vi "电源管理UI.vi"() -> ()   [LabVIEW 2016, in "PLC.lvlib"]
uses:
  PLC.lvlib
  <vilib>/Utility/miscctls.llb/LVPointTypeDef.ctl
  <vilib>/ptbypt/NI_PtbyPt.lvlib
panel:
  in  "电源控制":T1
  in  "副屏看门狗启用":u16(ring) caption="副屏看门狗启用：" items=["关闭", "打开"]
  in  "副屏看门狗设置":u16 caption="副屏看门狗设置："
  out "副屏看门狗计时":u16 caption="副屏看门狗计时："
  in  "主屏看门狗启用":u16(ring) caption="主屏看门狗启用：" items=["关闭", "打开"]
  in  "主屏看门狗设置":u16 caption="主屏看门狗设置："
  out "主屏看门狗计时":u16 caption="主屏看门狗计时："
  out "漏电报警累加值":u16 caption="漏电报警累加值："
  out "外部电源状态":u16(ring) caption="外部电源状态：" items=["正常", "异常"]
  out "当前报警状态":u16(ring) caption="当前报警状态：" items=["无报警"=0, "过压报警"=1, "欠压报警"=2, "过流报警"=4, "漏电报警"=8]
  out "通讯状态":u16(ring) caption="通讯状态：" items=["正常", "异常"]
  out "内部电源状态":u16(ring) caption="内部电源状态：" items=["异常", "正常"]
  out "过流报警累加值":u16 caption="过流报警累加值："
  out "欠压报警累加值":u16 caption="欠压报警累加值："
  out "过压报警累加值":u16 caption="过压报警累加值："
  out "当前漏电电流":dbl caption="当前漏电电流："
  out "当前电流":dbl caption="当前电流："
  out "当前电压":u16 caption="当前电压："
  # "s"
  # "s"
  # "s"
  # "s"
  # "mA"
  # "A"
  # "V"
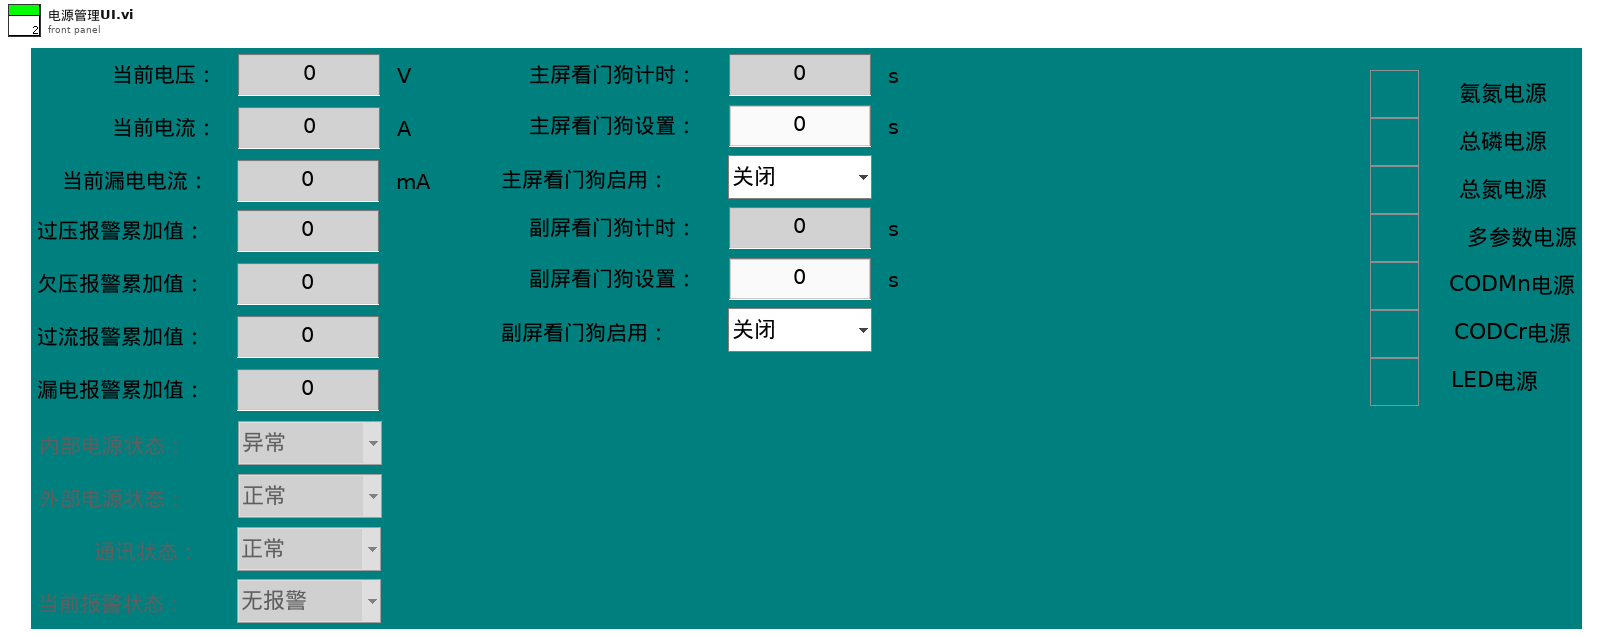
[diagram p1: front panel]
types:
  T1 = cluster{"氨氮电源":bool, "总磷电源":bool, "总氮电源":bool, "多参数电源":bool, "CODMn电源":bool, "CODCr电源":bool, "LED电源":bool}
  T2 = typedef "LVPointTypeDef.ctl" = cluster{"Horizontal":i16, "Vertical":i16}
  T3 = cluster{"R0":i16, "R1":i16, "R2":i16, "R3":i16, "R4":i16, "R5":i16, "R6":i16, "R7":i16, "R8":i16, "R9":i16, "R10":i16, "R11":i16, "R12":i16, "R13":i16, "R14":i16, "R15":i16, "R16":i16, "R17":i16, "R18":i16, "R19":i16, "R20":i16, "R21":i16, "R22":i16, "R23":i16, "R24":i16, "R25":i16, "R26":i16, "R27":i16, "R28":i16, "R29":i16, "R30":i16, "R31":i16, "R32":i16, "R33":i16, "R34":i16, "R35":i16, "R36":i16, "R37":i16, "R38":i16, "R39":i16}
  T4 = cluster{"R100":i16, "R101":i16, "R102":i16, "R103":i16, "R104":i16, "R105":i16, "R106":i16, "R107":i16, "R108":i16, "R109":i16, "R110":i16, "R111":i16, "R112":i16, "R113":i16, "R114":i16, "R115":i16, "R116":i16, "R117":i16, "R118":i16, "R119":i16, "R120":i16}
  T5 = cluster{"命令":string, "数据":cluster{"starting address":u16, "holding register values":u16[]}}
  T6 = cluster{"命令":string, "数据":cluster{"starting address":u16, "holding register value":u16}}
  T7 = cluster{"时间标识":timestamp, "设备":string, "日志信息":string}
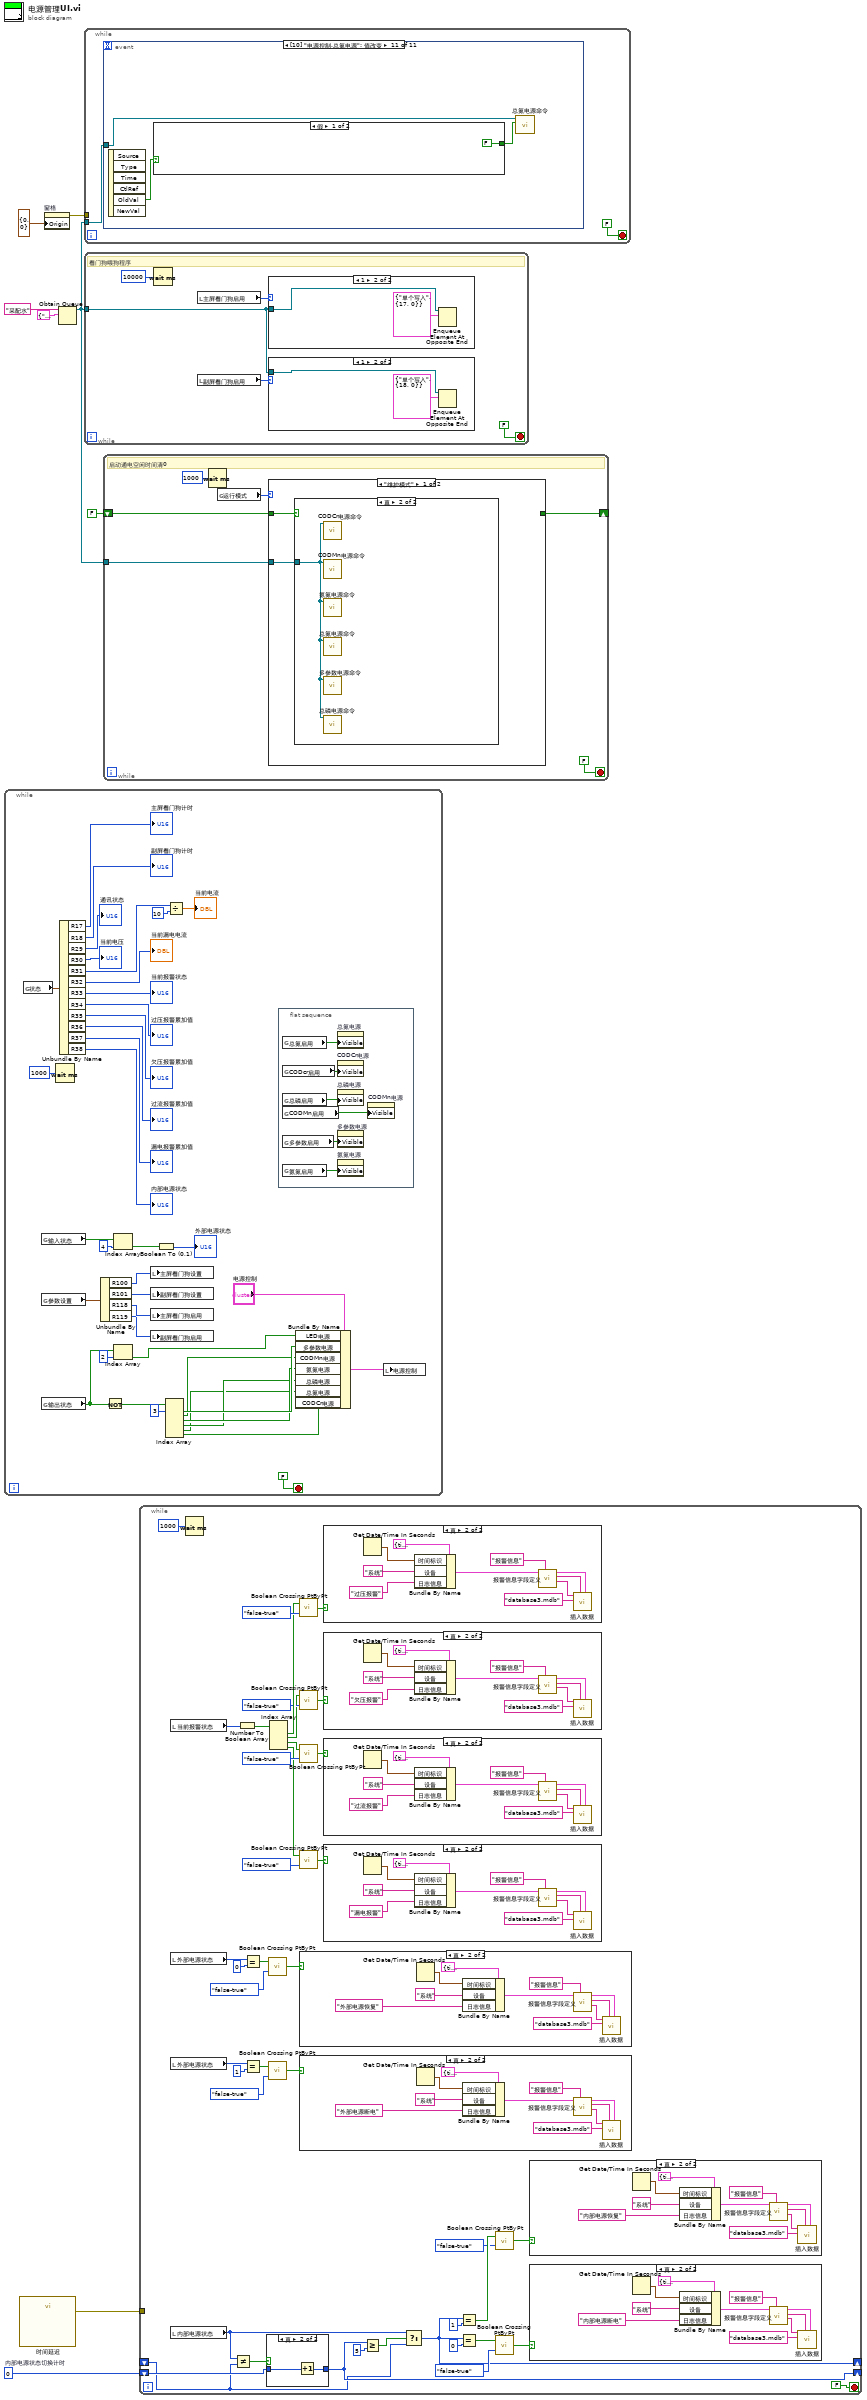
[diagram p0: block diagram]
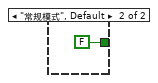
[diagram p14: hidden frame]
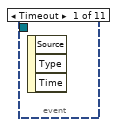
[diagram p15: hidden frame]
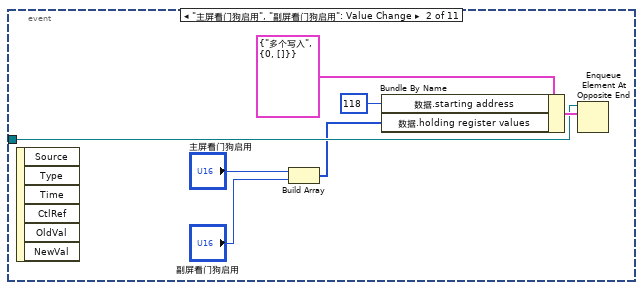
[diagram p16: hidden frame]
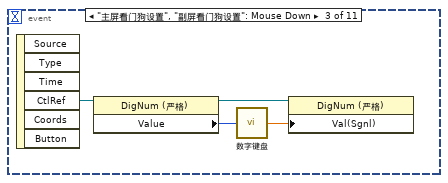
[diagram p17: hidden frame]
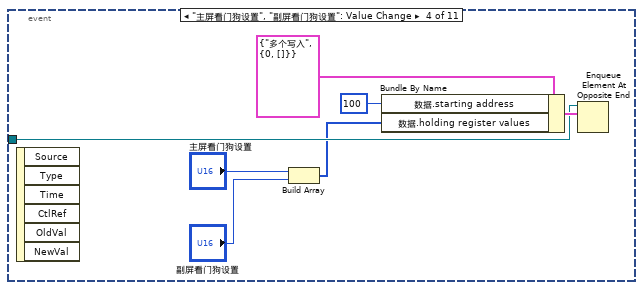
[diagram p18: hidden frame]
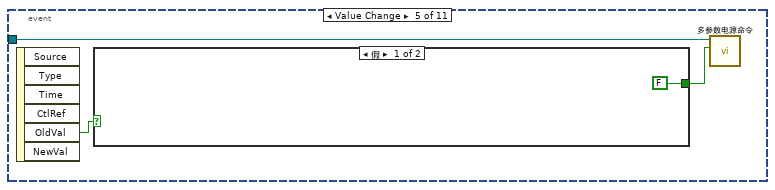
[diagram p19: hidden frame]
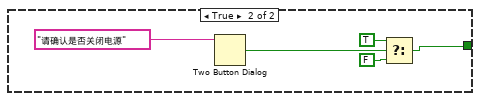
[diagram p20: hidden frame]
diagram:
  w1 = u16 0  # 内部电源状态切换计时
  n1 = while {
    stop <- FALSE stop-if-true
    n2 = global read "采配水全局变量.vi" "状态"() -> (w44:T3)
    n3 = global read "采配水全局变量.vi" "输入状态"() -> (w31:bool[])
    n4 = global read "采配水全局变量.vi" "参数设置"() -> (w25:T4)
    n5 = global read "采配水全局变量.vi" "输出状态"() -> (w19:bool[])
    n6 = Wait (ms)(milliseconds to wait=u32 1000 ("等待时间（毫秒）")) -> ()  [unwired: 1 out]
    n7 = Unbundle By Name(w44) -> ("R17"=→"主屏看门狗计时":i16, "R18"=→"副屏看门狗计时":i16, "R29"=→"通讯状态":i16, "R30"=→"当前电压":i16, "R31"=w41:i16, "R32"=→"当前漏电电流":i16, "R33"=→"当前报警状态":i16, "R34"=→"过压报警累加值":i16, "R35"=→"欠压报警累加值":i16, "R36"=→"过流报警累加值":i16, "R37"=→"漏电报警累加值":i16, "R38"=→"内部电源状态":i16)
    n8 = Unbundle By Name(w25) -> ("R100"=w24:i16, "R101"=w23:i16, "R118"=w22:i16, "R119"=w21:i16)
    n9 = Not(x=w19) -> (.not. x?=w45:bool[])
    n10 = Index Array(array=w31, index=4 ("索引")) -> (element=w29:bool)
    n11 = Index Array(array=w19, index=2 ("索引")) -> (element=w16:bool)
    n12 = local write "主屏看门狗设置"(w24) -> ()
    n13 = local write "副屏看门狗设置"(w23) -> ()
    n14 = local write "主屏看门狗启用"(w22) -> ()
    n15 = local write "副屏看门狗启用"(w21) -> ()
    n16 = Boolean To (0,1)(Boolean=w29) -> (0, 1=→"外部电源状态":i16)
    n17 = Index Array(array=w45, index #1=3 ("索引")) -> (element #1=w15:bool, element #2=w14:bool, element #3=w13:bool, element #4=w12:bool, element #5=w11:bool, element #6=w10:bool)  [unwired: 5 in]
    n18 = Divide(x=w41, y=i16 10) -> (x/y=→"当前电流":dbl)
    n19 = flat-sequence {
      frame #0 {
        n20 = global read "系统设置全局变量.vi" "总氮启用"() -> (w52:bool)
        n21 = global read "系统设置全局变量.vi" "CODcr启用"() -> (w49:bool)
        n22 = global read "系统设置全局变量.vi" "总磷启用"() -> (w48:bool)
        n23 = global read "系统设置全局变量.vi" "CODMn启用"() -> (w51:bool)
        n24 = global read "系统设置全局变量.vi" "多参数启用"() -> (w50:bool)
        n25 = global read "系统设置全局变量.vi" "氨氮启用"() -> (w53:bool)
        n26 = property on="总氮电源" class="Bool (严格)"("Visible"=w52) -> ()  [unwired: 2 in, 2 out]
        n27 = property on="CODCr电源" class="Bool (严格)"("Visible"=w49) -> ()  [unwired: 2 in, 2 out]
        n28 = property on="总磷电源" class="Bool (严格)"("Visible"=w48) -> ()  [unwired: 2 in, 2 out]
        n29 = property on="多参数电源" class="Bool (严格)"("Visible"=w50) -> ()  [unwired: 2 in, 2 out]
        n30 = property on="氨氮电源" class="Bool (严格)"("Visible"=w53) -> ()  [unwired: 2 in, 2 out]
        n31 = property on="CODMn电源" class="Bool (严格)"("Visible"=w51) -> ()  [unwired: 2 in, 2 out]
      }
    }
    n32 = Bundle By Name(cluster="电源控制", "LED电源"=w16, "多参数电源"=w15, "CODMn电源"=w14, "氨氮电源"=w13, "总磷电源"=w12, "总氮电源"=w11, "CODCr电源"=w10) -> (w9:T1)
    n33 = local write "电源控制"(w9) -> ()
  }
  n34 = call "时间延迟"() -> ("error out"=w3:errorcluster)  [unwired: 11 in]
  n35 = property on="窗格" class="Pane"("Origin"=T2 {"Horizontal"=0, "Vertical"=0} ("原点")) -> (error out=w5:errorcluster)  [unwired: 2 in, 1 out]
  n36 = Obtain Queue(name (unnamed)="采配水" ("名称（未命名）"), element data type=cluster{"命令":string, "数据":variant} {"命令"="", "数据"=variant}) -> (queue out=w2:refnum<queue>)  [unwired: 3 in, 2 out]
  n37 = while {
    tunnel: w2 -> [w54]
    tunnel: w5 -> [_]
    stop <- FALSE stop-if-true
    n38 = event shown="[10] \"电源控制.总氮电源\": 值改变" {
      selector: _ -> [_ _ _ _ _ _ _ _ _ _ _]
      dyn-events: _ -> [_ _ _ _ _ _ _ _ _ _ _]
      timeout: _ -> [_ _ _ _ _ _ _ _ _ _ _]
      tunnel: w54 -> [_ w59 _ w70 w76 w84 w94 w103 w112 w121 w130]
      event Timeout {
        n39 = event-data() -> ()  [unwired: 1 in, 3 out]
      }
      event "主屏看门狗启用", "副屏看门狗启用": Value Change {
        n40 = event-data() -> ()  [unwired: 1 in, 6 out]
        n41 = Build Array("主屏看门狗启用", "副屏看门狗启用") -> (w56:u16[])
        n42 = Bundle By Name(cluster=T5 {"命令"="多个写入", "数据"={"starting address"=0, "holding register values"=[]}} ("元素"), "数据.starting address"=u16 118, "数据.holding register values"=w56) -> (w60:T5)
        n43 = Enqueue Element At Opposite End(queue=w59, element=w60) -> ()  [unwired: 2 in, 3 out]
      }
      event "主屏看门狗设置", "副屏看门狗设置": Mouse Down {
        n44 = event-data() -> ("CtlRef"=w63:refnum<vi>)  [unwired: 1 in, 5 out]
        n45 = property class="DigNum (严格)"(reference=w63) -> (reference out=w65:refnum<vi>, "Value"=w66:u16)  [unwired: 1 in, 1 out]
        n46 = call "数字键盘.vi"("OldNumber"=w66) -> ("NewNumber"=w64:sgl)
        n47 = property class="DigNum (严格)"(reference=w65, "Val(Sgnl)"=w64) -> ()  [unwired: 1 in, 2 out]
      }
      event "主屏看门狗设置", "副屏看门狗设置": Value Change {
        n48 = event-data() -> ()  [unwired: 1 in, 6 out]
        n49 = Build Array("主屏看门狗设置", "副屏看门狗设置") -> (w67:u16[])
        n50 = Bundle By Name(cluster=T5 {"命令"="多个写入", "数据"={"starting address"=0, "holding register values"=[]}} ("元素"), "数据.starting address"=u16 100, "数据.holding register values"=w67) -> (w71:T5)
        n51 = Enqueue Element At Opposite End(queue=w70, element=w71) -> ()  [unwired: 2 in, 3 out]
      }
      event "电源控制.多参数电源": Value Change {
        n52 = event-data() -> ("OldVal"=w75:bool)  [unwired: 1 in, 5 out]
        n53 = case shown="假" w75 {
          tunnel: [FALSE ("T button?") w78] -> w74
          frame False {
          }
          frame True {
            n54 = Two Button Dialog(message="请确认是否关闭电源" ("消息")) -> (T button?=w81:bool)  [unwired: 2 in]
            n55 = Select(t=TRUE, s=w81, f=FALSE ("T button?")) -> (s? t:f=w78:bool)
          }
        }
        n56 = call "多参数电源命令.vi"("通电/断电"=w74, "队列"=w76) -> ()  [unwired: 9 in, 1 out]
      }
      event "电源控制.LED电源": Value Change {
        n57 = event-data() -> ("OldVal"=w85:bool)  [unwired: 1 in, 5 out]
        n58 = case shown="假" w85 {
          tunnel: [TRUE ("T button?") w87] -> w83
          frame False {
          }
          frame True {
            n59 = Two Button Dialog(message="请确认是否关闭电源" ("消息")) -> (T button?=w90:bool)  [unwired: 2 in]
            n60 = Select(t=FALSE, s=w90, f=TRUE ("T button?")) -> (s? t:f=w87:bool)
          }
        }
        n61 = call "LED电源命令.vi"("通电/断电"=w83, "队列"=w84) -> ()  [unwired: 9 in, 1 out]
      }
      event "电源控制.CODMn电源": Value Change {
        n62 = event-data() -> ("OldVal"=w93:bool)  [unwired: 1 in, 5 out]
        n63 = case shown="假" w93 {
          tunnel: [FALSE ("T button?") w96] -> w92
          frame False {
          }
          frame True {
            n64 = Two Button Dialog(message="请确认是否关闭电源" ("消息")) -> (T button?=w99:bool)  [unwired: 2 in]
            n65 = Select(t=TRUE, s=w99, f=FALSE ("T button?")) -> (s? t:f=w96:bool)
          }
        }
        n66 = call "CODMn电源命令.vi"("通电/断电"=w92, "队列"=w94) -> ()  [unwired: 9 in, 1 out]
      }
      event "电源控制.氨氮电源": Value Change {
        n67 = event-data() -> ("OldVal"=w102:bool)  [unwired: 1 in, 5 out]
        n68 = case shown="假" w102 {
          tunnel: [FALSE ("T button?") w105] -> w101
          frame False {
          }
          frame True {
            n69 = Two Button Dialog(message="请确认是否关闭电源" ("消息")) -> (T button?=w108:bool)  [unwired: 2 in]
            n70 = Select(t=TRUE, s=w108, f=FALSE ("T button?")) -> (s? t:f=w105:bool)
          }
        }
        n71 = call "氨氮电源命令.vi"("通电/断电"=w101, "队列"=w103) -> ()  [unwired: 9 in, 1 out]
      }
      event "电源控制.总磷电源": Value Change {
        n72 = event-data() -> ("OldVal"=w111:bool)  [unwired: 1 in, 5 out]
        n73 = case shown="假" w111 {
          tunnel: [FALSE ("T button?") w114] -> w110
          frame False {
          }
          frame True {
            n74 = Two Button Dialog(message="请确认是否关闭电源" ("消息")) -> (T button?=w117:bool)  [unwired: 2 in]
            n75 = Select(t=TRUE, s=w117, f=FALSE ("T button?")) -> (s? t:f=w114:bool)
          }
        }
        n76 = call "总磷电源命令.vi"("通电/断电"=w110, "队列"=w112) -> ()  [unwired: 9 in, 1 out]
      }
      event "电源控制.CODCr电源": Value Change {
        n77 = event-data() -> ("OldVal"=w120:bool)  [unwired: 1 in, 5 out]
        n78 = case shown="假" w120 {
          tunnel: [FALSE ("T button?") w123] -> w119
          frame False {
          }
          frame True {
            n79 = Two Button Dialog(message="请确认是否关闭电源" ("消息")) -> (T button?=w126:bool)  [unwired: 2 in]
            n80 = Select(t=TRUE, s=w126, f=FALSE ("T button?")) -> (s? t:f=w123:bool)
          }
        }
        n81 = call "CODCr电源命令.vi"("通电/断电"=w119, "队列"=w121) -> ()  [unwired: 9 in, 1 out]
      }
      event "电源控制.总氮电源": Value Change {
        n82 = event-data() -> ("OldVal"=w128:bool)  [unwired: 1 in, 5 out]
        n83 = case shown="假" w128 {
          tunnel: [FALSE ("T button?") w132] -> w129
          frame False {
          }
          frame True {
            n84 = Two Button Dialog(message="请确认是否关闭电源" ("消息")) -> (T button?=w135:bool)  [unwired: 2 in]
            n85 = Select(t=TRUE, s=w135, f=FALSE ("T button?")) -> (s? t:f=w132:bool)
          }
        }
        n86 = call "总氮电源命令.vi"("通电/断电"=w129, "队列"=w130) -> ()  [unwired: 9 in, 1 out]
      }
    }
  }
  n87 = while {
    tunnel: w2 -> [w140]
    stop <- FALSE stop-if-true
    # "看门狗喂狗程序"
    n88 = Wait (ms)(milliseconds to wait=u32 10000 ("等待时间（毫秒）")) -> ()  [unwired: 1 out]
    n89 = local read "主屏看门狗启用"() -> (w139:u16)
    n90 = local read "副屏看门狗启用"() -> (w138:u16)
    n91 = case shown="1" w139 {
      tunnel: w140 -> [_ w144]
      frame 0, Default {
      }
      frame 1 {
        n92 = Enqueue Element At Opposite End(queue=w144, element=T6 {"命令"="单个写入", "数据"={"starting address"=17, "holding register value"=0}} ("元素")) -> ()  [unwired: 2 in, 3 out]
      }
    }
    n93 = case shown="1" w138 {
      tunnel: w140 -> [_ w142]
      frame 0, Default {
      }
      frame 1 {
        n94 = Enqueue Element At Opposite End(queue=w142, element=T6 {"命令"="单个写入", "数据"={"starting address"=18, "holding register value"=0}} ("元素")) -> ()  [unwired: 2 in, 3 out]
      }
    }
  }
  n95 = while {
    tunnel: w2 -> [w149]
    shift-right: [w146] -> _
    shift-left: FALSE -> [w147]
    stop <- FALSE stop-if-true
    # "启动通电空闲时间清0"
    n96 = Wait (ms)(milliseconds to wait=u32 1000 ("等待时间（毫秒）")) -> ()  [unwired: 1 out]
    n97 = global read "系统设置全局变量.vi" "运行模式"() -> (w148:enum16{"维护模式", "常规模式", "应急模式", "质控模式"})
    n98 = case shown="\"维护模式\"" w148 {
      tunnel: w149 -> [w153 _]
      tunnel: w147 -> [w152 _]
      tunnel: [_ FALSE] -> w146
      frame "维护模式" {
        n99 = case shown="真" w152 {
          tunnel: w153 -> [_ w154]
          frame False {
          }
          frame True {
            n100 = call "CODCr电源命令.vi"("队列"=w154) -> ()  [unwired: 10 in, 1 out]
            n101 = call "CODMn电源命令.vi"("队列"=w154) -> ()  [unwired: 10 in, 1 out]
            n102 = call "氨氮电源命令.vi"("队列"=w154) -> ()  [unwired: 10 in, 1 out]
            n103 = call "总氮电源命令.vi"("队列"=w154) -> ()  [unwired: 10 in, 1 out]
            n104 = call "多参数电源命令.vi"("队列"=w154) -> ()  [unwired: 10 in, 1 out]
            n105 = call "总磷电源命令.vi"("队列"=w154) -> ()  [unwired: 10 in, 1 out]
          }
        }
      }
      frame "常规模式", Default {
      }
    }
  }
  n106 = while {
    tunnel: w3 -> [_]
    shift-right: [w161] -> _
    shift-left: w1 -> [w162]
    shift-right: [w156] -> _
    shift-left: _ -> [w157]
    stop <- FALSE stop-if-true
    n107 = local read "当前报警状态"() -> (w183:u16)
    n108 = local read "外部电源状态"() -> (w197:u16)
    n109 = local read "外部电源状态"() -> (w188:u16)
    n110 = local read "内部电源状态"() -> (w158:u16)
    n111 = Wait (ms)(milliseconds to wait=u32 1000 ("等待时间（毫秒）")) -> ()  [unwired: 1 out]
    n112 = Not Equal?(x=w158, y=w157) -> (x != y?=w167:bool)
    n113 = Number To Boolean Array(number=w183) -> (Boolean array=w182:bool[])
    n114 = Equal?(x=w197, y=u16 0) -> (x = y?=w195:bool)
    n115 = Equal?(x=w188, y=u16 1) -> (x = y?=w190:bool)
    n116 = case shown="真" w167 {
      tunnel: w162 -> [_ w209]
      tunnel: [_ w208] -> w161
      frame False {
      }
      frame True {
        n117 = Increment(x=w209) -> (x+1=w208:u16)
      }
    }
    n118 = call <vilib>:"Boolean Crossing PtByPt.vi"("direction"=enum16{"either", "false-true", "true-false"}."false-true", "input"=w195) -> ("crossing"=w193:bool)  [unwired: 1 in]
    n119 = call <vilib>:"Boolean Crossing PtByPt.vi"("direction"=enum16{"either", "false-true", "true-false"}."false-true", "input"=w190) -> ("crossing"=w192:bool)  [unwired: 1 in]
    n120 = Index Array(array=w182) -> (element #1=w180:bool, element #2=w174:bool, element #3=w173:bool, element #4=w170:bool)  [unwired: 4 in]
    n121 = call <vilib>:"Boolean Crossing PtByPt.vi"("direction"=enum16{"either", "false-true", "true-false"}."false-true", "input"=w180) -> ("crossing"=w179:bool)  [unwired: 1 in]
    n122 = call <vilib>:"Boolean Crossing PtByPt.vi"("direction"=enum16{"either", "false-true", "true-false"}."false-true", "input"=w174) -> ("crossing"=w178:bool)  [unwired: 1 in]
    n123 = call <vilib>:"Boolean Crossing PtByPt.vi"("direction"=enum16{"either", "false-true", "true-false"}."false-true", "input"=w173) -> ("crossing"=w175:bool)  [unwired: 1 in]
    n124 = call <vilib>:"Boolean Crossing PtByPt.vi"("direction"=enum16{"either", "false-true", "true-false"}."false-true", "input"=w170) -> ("crossing"=w172:bool)  [unwired: 1 in]
    n125 = case shown="真" w193 {
      frame False {
      }
      frame True {
        n126 = Get Date/Time In Seconds() -> (seconds since 1Jan1904=w278:timestamp)
        n127 = Bundle By Name(cluster=T7 {"时间标识"=timestamp(0 s since 1904-01-01), "设备"="", "日志信息"=""} ("data in"), "时间标识"=w278, "设备"="系统", "日志信息"="外部电源恢复") -> (w277:T7)
        n128 = call "报警信息字段定义.vi"("table输入"="报警信息", "data in"=w277) -> ("table输出"=w273:string, "columns"=w272:string[], "data out"=w271:T7)  [unwired: 7 in]
        n129 = call "插入数据.vi"("data"=w271, "columns"=w272, "database"="database3.mdb", "table"=w273) -> ()  [unwired: 7 in, 1 out]
      }
    }
    n130 = case shown="真" w192 {
      frame False {
      }
      frame True {
        n131 = Get Date/Time In Seconds() -> (seconds since 1Jan1904=w268:timestamp)
        n132 = Bundle By Name(cluster=T7 {"时间标识"=timestamp(0 s since 1904-01-01), "设备"="", "日志信息"=""} ("data in"), "时间标识"=w268, "设备"="系统", "日志信息"="外部电源断电") -> (w267:T7)
        n133 = call "报警信息字段定义.vi"("table输入"="报警信息", "data in"=w267) -> ("table输出"=w263:string, "columns"=w262:string[], "data out"=w261:T7)  [unwired: 7 in]
        n134 = call "插入数据.vi"("data"=w261, "columns"=w262, "database"="database3.mdb", "table"=w263) -> ()  [unwired: 7 in, 1 out]
      }
    }
    n135 = case shown="真" w179 {
      frame False {
      }
      frame True {
        n136 = Get Date/Time In Seconds() -> (seconds since 1Jan1904=w248:timestamp)
        n137 = Bundle By Name(cluster=T7 {"时间标识"=timestamp(0 s since 1904-01-01), "设备"="", "日志信息"=""} ("data in"), "时间标识"=w248, "设备"="系统", "日志信息"="过压报警") -> (w247:T7)
        n138 = call "报警信息字段定义.vi"("table输入"="报警信息", "data in"=w247) -> ("table输出"=w243:string, "columns"=w242:string[], "data out"=w241:T7)  [unwired: 7 in]
        n139 = call "插入数据.vi"("data"=w241, "columns"=w242, "database"="database3.mdb", "table"=w243) -> ()  [unwired: 7 in, 1 out]
      }
    }
    n140 = case shown="真" w178 {
      frame False {
      }
      frame True {
        n141 = Get Date/Time In Seconds() -> (seconds since 1Jan1904=w238:timestamp)
        n142 = Bundle By Name(cluster=T7 {"时间标识"=timestamp(0 s since 1904-01-01), "设备"="", "日志信息"=""} ("data in"), "时间标识"=w238, "设备"="系统", "日志信息"="欠压报警") -> (w237:T7)
        n143 = call "报警信息字段定义.vi"("table输入"="报警信息", "data in"=w237) -> ("table输出"=w233:string, "columns"=w232:string[], "data out"=w231:T7)  [unwired: 7 in]
        n144 = call "插入数据.vi"("data"=w231, "columns"=w232, "database"="database3.mdb", "table"=w233) -> ()  [unwired: 7 in, 1 out]
      }
    }
    n145 = case shown="真" w175 {
      frame False {
      }
      frame True {
        n146 = Get Date/Time In Seconds() -> (seconds since 1Jan1904=w228:timestamp)
        n147 = Bundle By Name(cluster=T7 {"时间标识"=timestamp(0 s since 1904-01-01), "设备"="", "日志信息"=""} ("data in"), "时间标识"=w228, "设备"="系统", "日志信息"="过流报警") -> (w227:T7)
        n148 = call "报警信息字段定义.vi"("table输入"="报警信息", "data in"=w227) -> ("table输出"=w223:string, "columns"=w222:string[], "data out"=w221:T7)  [unwired: 7 in]
        n149 = call "插入数据.vi"("data"=w221, "columns"=w222, "database"="database3.mdb", "table"=w223) -> ()  [unwired: 7 in, 1 out]
      }
    }
    n150 = case shown="真" w172 {
      frame False {
      }
      frame True {
        n151 = Get Date/Time In Seconds() -> (seconds since 1Jan1904=w218:timestamp)
        n152 = Bundle By Name(cluster=T7 {"时间标识"=timestamp(0 s since 1904-01-01), "设备"="", "日志信息"=""} ("data in"), "时间标识"=w218, "设备"="系统", "日志信息"="漏电报警") -> (w217:T7)
        n153 = call "报警信息字段定义.vi"("table输入"="报警信息", "data in"=w217) -> ("table输出"=w213:string, "columns"=w212:string[], "data out"=w211:T7)  [unwired: 7 in]
        n154 = call "插入数据.vi"("data"=w211, "columns"=w212, "database"="database3.mdb", "table"=w213) -> ()  [unwired: 7 in, 1 out]
      }
    }
    n155 = Greater Or Equal?(x=w161, y=u16 5) -> (x >= y?=w159:bool)
    n156 = Select(t=w158, s=w159, f=w157) -> (s? t:f=w156:u16)
    n157 = Equal?(x=w156, y=u16 1) -> (x = y?=w166:bool)
    n158 = Equal?(x=w156, y=u16 0) -> (x = y?=w185:bool)
    n159 = call <vilib>:"Boolean Crossing PtByPt.vi"("direction"=enum16{"either", "false-true", "true-false"}."false-true", "input"=w166) -> ("crossing"=w164:bool)  [unwired: 1 in]
    n160 = call <vilib>:"Boolean Crossing PtByPt.vi"("direction"=enum16{"either", "false-true", "true-false"}."false-true", "input"=w185) -> ("crossing"=w187:bool)  [unwired: 1 in]
    n161 = case shown="真" w164 {
      frame False {
      }
      frame True {
        n162 = Get Date/Time In Seconds() -> (seconds since 1Jan1904=w206:timestamp)
        n163 = Bundle By Name(cluster=T7 {"时间标识"=timestamp(0 s since 1904-01-01), "设备"="", "日志信息"=""} ("data in"), "时间标识"=w206, "设备"="系统", "日志信息"="内部电源恢复") -> (w205:T7)
        n164 = call "报警信息字段定义.vi"("table输入"="报警信息", "data in"=w205) -> ("table输出"=w201:string, "columns"=w200:string[], "data out"=w199:T7)  [unwired: 7 in]
        n165 = call "插入数据.vi"("data"=w199, "columns"=w200, "database"="database3.mdb", "table"=w201) -> ()  [unwired: 7 in, 1 out]
      }
    }
    n166 = case shown="真" w187 {
      frame False {
      }
      frame True {
        n167 = Get Date/Time In Seconds() -> (seconds since 1Jan1904=w258:timestamp)
        n168 = Bundle By Name(cluster=T7 {"时间标识"=timestamp(0 s since 1904-01-01), "设备"="", "日志信息"=""} ("data in"), "时间标识"=w258, "设备"="系统", "日志信息"="内部电源断电") -> (w257:T7)
        n169 = call "报警信息字段定义.vi"("table输入"="报警信息", "data in"=w257) -> ("table输出"=w253:string, "columns"=w252:string[], "data out"=w251:T7)  [unwired: 7 in]
        n170 = call "插入数据.vi"("data"=w251, "columns"=w252, "database"="database3.mdb", "table"=w253) -> ()  [unwired: 7 in, 1 out]
      }
    }
  }
